vi "Write Glass Data.vi"(4 "DBL Array":dbl[][](array[numeric]), 6 "Waveforms":waveform(dbl)[](array[waveform]), 8 "error in":errorcluster, 11 "Glass Data in":variant) -> (0 "error out":errorcluster, 3 "Glass Data out":variant)   [LabVIEW 2015, in "Exposure Process.lvlib"]
uses:
  Exposure Process.lvlib
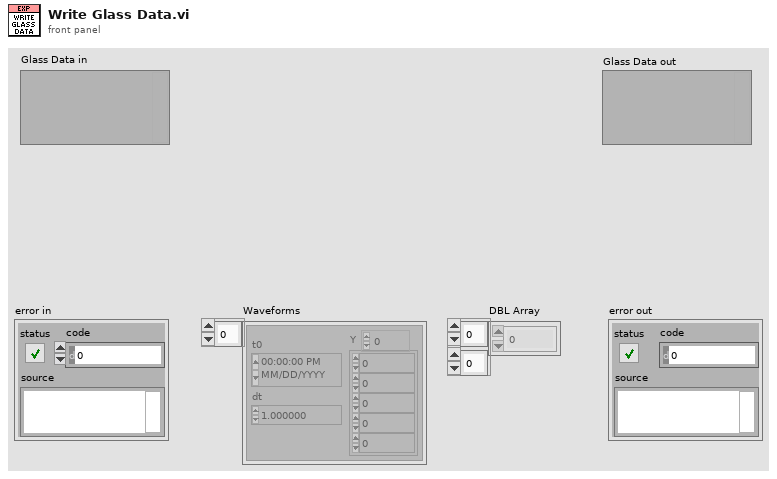
[diagram p1: front panel]
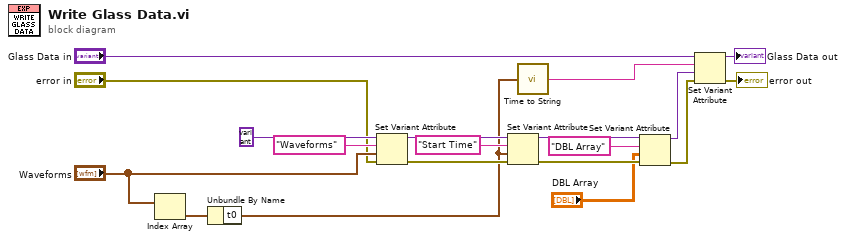
[diagram p0: block diagram]
diagram:
  n1 = Index Array(array="Waveforms") -> (element=w18:waveform(dbl))  [unwired: 1 in]
  n2 = Unbundle By Name(w18) -> ("t0"=w7:timestamp)
  n3 = Set Variant Attribute(Variant=variant, name="Waveforms", value="Waveforms", error in="error in") -> (Variant out=w15:variant, error out=w14:errorcluster)  [unwired: 1 out]
  n4 = Set Variant Attribute(Variant=w15, name="Start Time", value=w7, error in=w14) -> (Variant out=w12:variant, error out=w11:errorcluster)  [unwired: 1 out]
  n5 = call "Time to String.vi"("Time Stamp"=w7) -> ("date/time string"=w6:string)
  n6 = Set Variant Attribute(Variant=w12, name="DBL Array", value="DBL Array", error in=w11) -> (Variant out=w4:variant, error out=w5:errorcluster)  [unwired: 1 out]
  n7 = Set Variant Attribute(Variant="Glass Data in", name=w6, value=w4, error in=w5) -> (Variant out=→"Glass Data out":variant, error out=→"error out":errorcluster)  [unwired: 1 out]
